vi "Update Card.vi"(8 "error in (no error)":errorcluster, 11 "BME_DG_G05_Chnl in":refnum<class "BME_DG_G08_Chnl.lvclass">) -> (0 "error out":errorcluster, 3 "BME_DG_G05_Chnl out":refnum<class "BME_DG_G08_Chnl.lvclass">)   [LabVIEW 2009, in "BME_DG_G08_Chnl.lvclass"]
uses:
  BME_DG_G08_Chnl.lvclass
  BME_DG_G08_Chnl.lvclass/BME_DG_G08_Chnl.ctl
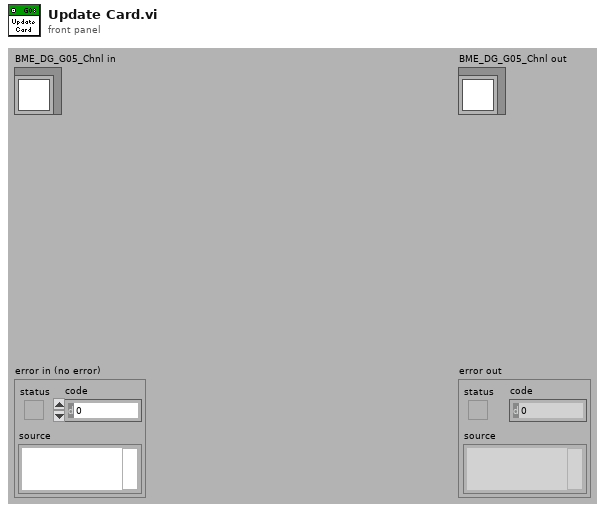
[diagram p1: front panel]
types:
  T1 = cluster{"Channel":u32, "Fire First (µs)":dbl, "Pulse Width (µs)":dbl, "Output Modulo":u32, "Output Offset":u32, "Go Signal":u32, "Polarity":bool, "Terminate":bool, "Disconnect (E,F)":bool, "Onto MsBus (E,F)":bool, "Input Positive (E,F)":bool}
  T2 = typedef "ChnlSettings.ctl" = cluster{" Delay (µs)":dbl, "On? (false)":bool, "PositiveVoltage?(true)":bool, "50OhmTerminated? ":bool, "25OhmOutput?":bool}
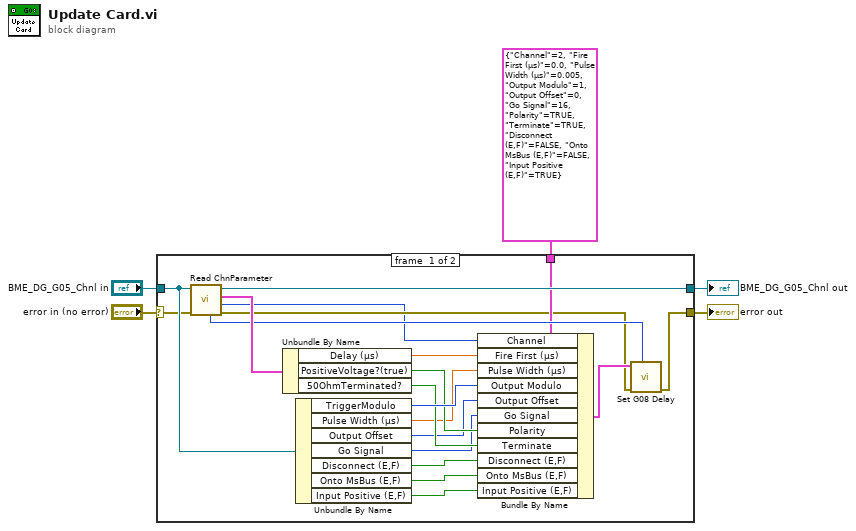
[diagram p0: block diagram]
diagram:
  n1 = case shown="No Error" "error in (no error)" {
    selector: "error in (no error)" -> [w22 w27]
    tunnel: [w18 w27] -> w2
    tunnel: [w25 w26] -> w4
    tunnel: "BME_DG_G05_Chnl in" -> [w23 w26]
    tunnel: T1 {"Channel"=2, "Fire First (µs)"=0.0, "Pulse Width (µs)"=0.005, "Output Modulo"=1, "Output Offset"=0, "Go Signal"=16, "Polarity"=TRUE, "Terminate"=TRUE, "Disconnect (E,F)"=FALSE, "Onto MsBus (E,F)"=FALSE, "Input Positive (E,F)"=TRUE} ("Settings") -> [w20 _]
    frame #0 {
      n2 = call-dynamic "Read ChnParameter.vi"("error in (no error)"=w22, "BME_DG_Chnl in"=w23) -> ("error out"=w17:errorcluster, "Nr"=w16:i32, "ChnParemater"=w24:T2, "BME_DG_Chnl out"=w25:refnum<class "BME_DG_G08_Chnl.lvclass">, "DG Nr"=w21:i32)  [unwired: 4 in, 1 out]
      n3 = Unbundle By Name(w24) -> ("Delay (µs)"=w15:dbl, "PositiveVoltage?(true)"=w12:bool, "50OhmTerminated?"=w13:bool)
      n4 = Unbundle By Name(w23) -> ("TriggerModulo"=w14:i32, "Pulse Width (µs)"=w11:dbl, "Output Offset"=w10:u32, "Go Signal"=w9:u32, "Disconnect (E,F)"=w8:bool, "Onto MsBus (E,F)"=w7:bool, "Input Positive (E,F)"=w6:bool)
      n5 = Bundle By Name(cluster=w20, "Channel"=w16, "Fire First (µs)"=w15, "Pulse Width (µs)"=w11, "Output Modulo"=w14, "Output Offset"=w10, "Go Signal"=w9, "Polarity"=w12, "Terminate"=w13, "Disconnect (E,F)"=w8, "Onto MsBus (E,F)"=w7, "Input Positive (E,F)"=w6) -> (w19:T1)
      n6 = call "Set G08 Delay.vi"("DG Number"=w21, "error in (no error)"=w17, "Settings"=w19) -> ("error out"=w18:errorcluster)  [unwired: 8 in]
    }
    frame #1 {
    }
  }
  "error out" <- w2
  "BME_DG_G05_Chnl out" <- w4
